vi "11_1.vi"() -> ()   [LabVIEW 2018]
uses:
  <userlib>/_OpenG.lib/array/array.llb/Search 1D Array (String)__ogtk.vi
panel:
  out "Occupied Seats":i32
  in  "Input":string="LLLLLLLLLLLLLLLLLLLLLLLLL.LLLLL..LLLLLLLLLLLL.LLL..LLLLLLLLLLLLLL.LL.LLLLL.LLLLLLLLL.LLLLLLLLLLLLL\nLLLLLLL.LLLLLLL.LLLLLLLLL.LLLLL.LLLL.LLLLLLLL.LLLLLLLLL.LLLL.LLLLLLLLLLLLLLLLLLLLLL..LLLLLLL..LLLL\nLLLLLL.LLLLLLLLLLLLLLLLLL.LLLLL.LLLLLLLLL.LLL.LLLLLLLLLLLLLL.LLLLLLL..LLLLLLLLLLLLLLLLLLLLLL.LLLLL\nLLLLLLL.LLLLLLLLLLLLLLLLLLLLLLL.LLLL.LLLLLLLLLLLLLLLLLLLL.LLLLLLLLLLLLLLL..LLLLLLLLL.LLLLLLL..LLLL\n.LLL.LL.LLLLLLL.LLLLLLLLL.LLLLLLLLLLLLLLLLLLLLLLLLLLLLLLLLLL.LLLLLLL.LLLLL.LLLLLLLLL.LLLLLLLLLLLLL\nLL.LLLL.LLLLLLLLLLLLLLLLL.LLLLL.LLLL.LLLLLLLLLLLLL.LLL.LLLLLLLLLLLLL.LLLLLLLLLLLLLLL.LLLLLLL.LLLLL\n......L........LLL....L.L......L.LL...L.....L.LL..L..L..L..LLL..LL......L...L.LL.L.L....L.........\nLLLLLLL.LLLLLLL.LLLLLLLLL.LLLLLLLLLL.LLLLLLLLL.LLL.LLLLLLLLL.L.LLLLL.LLLLL.LLLLLLLLL.LLLLLLL.LLLLL\nLLLLLLLLLLLLLLL.LLLLLLLLL.LLLLL.LLLL.LLLLLLLLLLLLLLLLLLLLLLL.LLLLLLL.LLLLL.LLLLLLLLLLLLLLLLL.LLLLL\nLLLLLLL.LLLLLLL.LLLLLLLLL.LLLLL.LLLL.LLLLLLLL.LLLL.LLLLLL.LL.LLLLLLL.LLLLLLLLLLLLLLL.LLLLLLL.LLLLL\nLLLLLLLLLLLLLLL.LLLLLLLLL.LLLLL.LLLL..LLLLLLL.LLLLLLLLLLLLLL.LLL.LLL..LLLL.LLLLLLLLL.LLLLLLL.LLLLL\nLLLLLLL.LLL.LLLLLLL.LLLLL.LLLLL.LLLL.LLLLLLLL.LLLL.LLLLLLLLLLLL.LLLL.L.LLL.LLLLLLLLLLLLLLLLL.LLLLL\nLLLLL.L.LLLLLLL.LLLLLL.LL.LLLLL.LLLL.LLLLLLLL.LLLL.LLLLLLLLL.L.L..LLLLLLL.LLLLLLLLLL.LLLLLLLLLLLLL\n.L....LLLL.LL.LL..L.L.L.L.LL..L..L.LLLLLL.L.LLLL.L.L..LL...L..L..LLL.....L........LL.L..L..L..L..L\nLLLLLLL.LLLLLLL.LLLLL.LLL.LLLLLLLLLL.LLLLL.LLLLLLL.LLLLLLLLLLLLLLLLLLLLLLL.LLLLLLLLL.LLLLLLLLLLLLL\nLLLLLLLLLLLLLLLLLL.LLLLLLLLLLLL..LLLLLLLLLLLL.LLLL.LLLLLLLLL.LLLLLLL.LLLLLLLLLLLLLLLLLLLLLLL.LLLLL\nLLLLLLL.LL.LLLL.LLLLLLLLLLLLLL.LLLLLLLL.LLLLLLLLLLLLLLLLLLLL.LLLLLLL.LLLLLLLLLLLLLLLLLLLLLLL.LLLLL\nLLLLLLL.LLLLLLL.LLLLLLLLL.LLLLL.LLLLLLLLLLLLL.LLLLLLLLLLLLLLLLLLLLLL.LLLLL.LLLLLLLLL.LLLLLLL.LLL.L\nLLLLLLLLLLLLLLL.LLLLLLLLL.LLLLLLLLLL.LLLLLLLLLLLLL.LLLLLLLLL.LLLLLLL.LLLLLLLL.LLLLLLLLLLL.LL.LLLLL\n.....L..L...L.L.L..........L..LLLL....L..L.L..LLLL...L..L....L.LL.L....L.L.L....LL.L..L......LLL.L\nLLLLLLL.LLLLLLL.LLLLLLLLLLLLLLLLLLLL.LLLLLLLLLLLLL.LLLLLLLLLLLLLLLLL.LLLLL.LL.LLLLLL.LL.LLLL.LLLLL\nLLLLLLL.L.LLLLLLLLLL.LLLL.L.LLLLLLLLLLLLLLLLLLLLLL.LLLLLLLLL.LLLLLLLLL.LLLLLLLLLLLLL.LLLLLLLLLLLLL\nLLLLLLL.LLLLLLL.LLLLLLLLL.LLLLL.LLLLLLLLLLLLL.LLLL.LLLLLLLLLLLLLLLLL.LLLLLLLLLLLL.LLLLLLLLLL.LLLLL\nLLLLLLL.LLLLLLLLLLLLLLLLL.LLLLL.L.LL.LLLLLLLLLLLLL.LLLLLLLLL.LLLL.LLLLLLLLLLLLLLL.L..LLLLLLLLLLL.L\nLLLLLLL.LLLLLLLLLLLLLLLLL.LLLLLLLLLL.LLLLLL.L.LLLL.L.LLLLLLLLLLLLLLL.LLLLLLLLLLLLL.L.LLLLLLLLLLLLL\nLLLLLLLLLLLLLLL.LLLLLL.LL.LLLLL.LLLLLLLLLLLLLLLLLLLLLLLLLLLL.LLLLLLL.LLLLL.LLLLLLLLL.LLLLLLL.LLLLL\nLLLLLLL.LL.LLLLLLLL.LLLLL.LLLLL.LLLL.LLLLLLLL.LLLLLLLLLLLLLL.LLLLLLL.LLLLL.LLLLLLL.L.LLLLLLL.LLLLL\nL.LLLLL.LLLLLLL.LLLLLLLLL.LLLLL.LLLLLLLLLLLLL.LLLLLLLLLLLLLL.LLLLLLL.LLLLLLLLLLLLLLL.LLLLLLLLLLLLL\nLLLLLLLLLLLLLLLLLLLLLLLLL.LLLLL.LLLLLLLLLLLLLLLLLL.LLLL.LLLL.LLLLLLL.LLLLLLLLLLLLLLLLLLLLLLLL.LLLL\n..L...L...L......L.LLLL.....LLL.L.LLLLLL.L.L.L..L.L.......L.L..L...L.L.L....LL...L.LL......LL.L.L.\nLLLLLLL.LLLLLLL.L.LLLLLLL.LLLLL.LLL.LLLLLLLLL.LLLLLLLLLLLLLL.LLLLLLL.LLLLL.LLLLLLLLL.LLLLLLL.LLLLL\nLLLLLLL.LLLLLLL.LLLLLLLLLLLLLLL.LLLLLLLLLLLLL..LLL.LLLLLLLLLLLLLLLLL.LLLLL.LLLLLLLLL.LLLLLLL.LLLLL\nLLLLLLL.LLLLLLLLLLLLLLLLL.LLLLL.LLLLLLLLLLLLLLLLLL.LLLLLLLLL.LLLLLLL.LLL.L.LLLLL.LLLLLLLLLLL.LLLLL\nLLLLLLL.LLLLLLL.LL.LLLLLL..LLLL.LLLLLLLLLLLLLLLLLLLLLLLLLLLLLLLLLLLL.LLLLL..LLLLLLLL.LLLL.LL.LLLLL\nLL.LLLL.LLLLLLLLL.LLLLLLL.LLLLLLLLLLLLLLLLLLLLLLLL.L.LLLLL.LLLLLLLLLLLLLLLLLLLLLLL.L.LLLLLLL.LLLLL\nLLLLLLL.LLLLLLL.LLLLLLLLL.LLLLL.LLLL.LLLLLLLL.LLLL.LLLLLL.LL.LLLLL.L.LLLLL.LLLLLLLLLLLLLLLLLLLLLLL\nLLLLLLL.LLL.LLL.LLLLLLLLLLLLLLL.LLLL.LLLLLLLL.LLLLLLLLLLLL.LLLLLLLLLLLLLLL.LLLLLLLLL.LLLLLLL.LLLLL\nL.L.......L.L....LL......LL.LL...LL..L...........L.....LLL....L..LL.LL.L.L.LL.......L.L...L....L..\nLLLLLLL.LLLLLLLLLLLLLLLLL.LLLLL.LLLL.LLLLLLLLLLLLL.LLLLLLLLL.LLLLLLL.LL.LL.LLLLLLLLLLLLLLLLL.LLL.L\nLLLLLLL.LLLLLLLLLLLLLLLLLLLLLLL.LLLL.LL.LLLLLLLLLL.LL.LLLLLL.LLLLLLLLLLLLL.LLLLLLLLLLLLLLLLLLLLLLL\nLLLLLLL.LLLLLLL.LLLLLLLLL.LLLLL.LLLL..LLLLLLLLLLLL.LLLLLLLLLLLLLLLLL.L..LL.LLL.LLLLLLLLLLLLLLLLLLL\nLLLLLLLLLL.LLLLLLLLLLLLLLLLLLLL.LLLL.LLLLLLLLLLLLL.LLLLLLLLLLLLLLLLLLLLLLL.LLLLLLLLL.LLLLLLL.LLLLL\nLLLLLLLLLL.LLLL.LLLLLLL.LLL.LLLLLLLL.LLLLLLLLLLLLL.LLLLLLLLL.LLLLLLLLLLLLLLLLLLLLLLLLLLLLLLL.LLLLL\nL.LLLLLLLLLLLLL.LL.LLLLLL.LLLLL.LLLL.LLLLLLLL.LLLLLLLLLLL.LL.LLLL.LLLLLLLLLL.LLLLLLL.LLLLLLL.LLLLL\n...LL.L..LL...L.......L.LL.......LL.LLL.L.LLL...L..LLL.L...L.......LL.LL.LL.L..LL........L.......L\nLLLLLLL.LLLLLLL.LLLLLLLLL.LLLLL.LLLL.LLLLLLLL.LLLLLLLLLLLLLL.LLLLLLL.LLLLL.LLLLLLLLLLLLLLLLL.LLLLL\nLLLLLLL.LLLLLLL.LLLLLLLLLLLLLLL.LLLL.LLLLLLLL.LLLLLLLLL.LLLL.LLLLLLL.LLLLL.LLLLLLLLLLLLLLLLLLLLLLL\nLLLLLLL.LLLLLLLLLLLLLLLLL.LLLLL.LLLLLLLLLLLLL.LLLL.LLLLLLLLL.LLLLL.L..LLLL.LLLLLLLLL.LLLL.LLLLLLLL\nLLLLLLLLLLLLLLL.LLLLLLLLLLLLLLL.LLLL.LLLLLLLL.LLLL..LLLLLLLLLLLLLLL..LL.LL.L.LLL.LLL.LLLLLLL.LLLLL\nLLLLL..LLLL.LLLLLLLLLLLLL.LLLLLLLL.L.LLLLLLLL.LLLL.LLLLLLLLL.L.LLL.LLLLLLL.LLLLLLLLL.LLLLLLLLLLLLL\nLLLLLLLLLLLLLLLLLLLLLLLLLLLLLLL.LLLL.LLLLLLLL.LLLL.LLLLLLLLLLLLLLLLLLLLL.L.LLLLLLLLL.LLLLL.L.LLLLL\n.LLLLLL.LLLLLLL..LLLLLLLL.LLLLLLLLLLLLLLLLLLL.LLLLLLLLLLLLLLLLLLLLLLLLLLLL.LLLLLLLLL.LLLLLLL.LLLLL\nLLLLLLL.LLLLLLLLLLL.LLLLLLLLLLLLLLL.LLLLLLLLLLLLLLLLLLLLLLLL.LLLLLLL.LLLLLLLLLLLLLLLLLLLLLLL.LLLLL\n..LL....L..........LL..L....L.LL...L.L...L.L...LLL..LL....LL.L.L.LLLL...L.L.......L.....LL........\nLLLLLLL.LLLLLLL.LLLLLLLLLLLLLLLLLLLL.LLLLLLLL.LLLLLLLLLLLLLL.LLLLLLLLLLLLLLLLLLLLLLL.LLLLLLL.LL.L.\nLLLLLLL.LLLL.LL.LLL.LLLLL.LLLLL.LLLL.LLLLLLL.LLLLL.LLLLLLLLLLLLLLLLL.LLLLLLLLLLLLLLL.LL.LLLLLLL.LL\nLL.LLLLLLLLLL.LLLLLLLLLLL.LLLLL.LLLL.LLLLLLLL.LLLL.LLLLLLLLL.LLL.LLL.LLLLL.LLLLLLLLL.LLLLLLL.LLLLL\nLLLLLLLLLLLLLLLL.LLLLLLLLLLLLLL.LLLL.LLLLLLLL.LLLLLLLLLLLLLL.LLLLLLL.LLLLL.LLLLLLLLL.LLLLLLL.LLLL.\nLLLLLLLLLLLLLLL.LLLLLLLL.LLLLLL.LLLL.LLLLLLLLLLLLL.LLLLLLLLL.LLL.LLL.L.LLLLLLLLLLLLLLLLLLLLL.LLLLL\nLLLLLLL.LLLLLLL.LLLLLLL.L.LLLLL.LLLL.LLLL.LLL.LLLLLLLLLL.LLLLLLLLLLL.LLLLL.LLLLLLLLL.LLLLLLL.LLL.L\nLLLLLLL.LLLLLLL.LLLLLLLLLLLLLLL.LLLL.L.LLLLLLLLLLL.LLLLLLLLL.LL.LLLL.LLLLLLLLLLLLLLL.LLLLLLLLLLLLL\nLLL.LLL.L.LLLLL.LLLLLLLLL.LLLLL.LLLL.LLLLLLLL.LLLL.LLLLLLL.L.LLLLLLLLL.LLL.LLLLLLLLLLLLLLLLLLLLLLL\n..LLL.LL.....LL...LL..L..LLL...........LL...........L.....L.......L..LLLLL......L......LL..L...L.L\nLLLLLLL.LLLLLLL.L.LLLLLLLLLL.LL.LLLL.LLLLLLLLLLLLL.LLLLLLL.L.LLLLLLLLLLLLLLLLLLLLLLLLLLLLLLL.LLLLL\nLLLLLLLLLLLLLLL.LL..LL.LLLLLLLL.LLLL.LLLLLLLLLLLLLLLLLLLLLLLLLLLLLLL.LLLLL.LLLLLLLLL.LLL.LLL.LLLLL\nLLLLLLL.LLLLLLL.LLLLLLLLL.LLLLL.LLLLLLLLLLLLL.LLLL.LLLLLLLLL.LLLLLLL..LLLL.LLLLLLLLLLLLLLLLLLLLLLL\nLLLLLLLLLLLL.LLLLLLLLLLLLLLLLLL.LLLLLLLLLLLLL.LLLL.LLLLLLLLL.LLLLLLLLL.LLLLLLLLLLLLLLLLLLLLL.LLLLL\nLLLLLLLLLLLLLLL.LLLLLLLLL.LLLLL.LLLLLLLLLLLLL.LLLLLLLLL.LLLL.LLLLLLL.LLLLLLLLLLLLLLL.LLLLLLLLLLLLL\nLLLLLLL.LLLLLLL.LLLLLLLLL.LLLLL.LLLL.LL.LLLLL.LLLL.LLLLLLLLL.LLLLLL.LLLLLL.LLLLLLLLL.LLLLLLL.L.LLL\nLLLLLLLLLLLLLLLLLLLLLLLLLLLLLLLLLLLL.LLLLLLLL.LLL..LLLLLLLLL.LLLLLLL.LLLLL.LLLLLLLLL.LLLLLLL..LLLL\nLLLLLLL.LLLLLLLLL.LLLLLLLLLLLLL.LLLL.LLLLLLLLLLLLL.LLLLLLLLL.LLLLLLLLLLLLL.LLLLLLL.LL.LLLLLLLLLLLL\nLLLLLLLLLLLLLLL.LLLLLLLLLLLLLLL.LLLL.LLLLLLLL.LLLL.LLLLLLLLL.LLLLLLL.LLLL..LLLLLLLLLLLLLLLLL.LLLLL\n.......L...LLL.L....L.LL......L.L...L...LL.LL...L...L..L.L.LL.........L.L..L.L.L.......L..L.....L.\nLLLLLLLLLLLLLLL.LLLLLLLLL.LLLLLLLLLL.LLLLLLL..LLLLLLLLLLLLL..LLLLL.LLLLLLL.LLLLLLLLL.LLLLLLLLLLLLL\nLLLLLLLLLLLLLLL.LLLLLLLLL.LLLLL.LLLL.LLLLLLLLLLLLL.LLLLLLLLL.LL.LLLLLLLLLL.LLLLLLLLLLLLLLLLL.LLLLL\nLLLLLLL.LLLLLLL.LLLLLLLLLLLLLLLLLLLLLLLLLLLLL.LL.LLLLLLLLLLLLLLLLL.L.LLLLL.LLLLLLLLL.LLLLLLL.LLLLL\nLLLLLLL.LLLLLLL.LLLLLLLLL.LLLLL.LLLLLLLLLLLLLLLLLL.LLLLL.LLL.LLLLLLLLLLLLL.L.LLLLLLL.LLLLLLLLLLLLL\nLLLLLLL.LLL.LLL.LLLLLLLLL.LLLLL.LLLLLLLLLLLLL.LLLL.LLLLLLLLL.LLLLLLL.LLLLL.LLLLLLLLLLLLLLLLL.LLLLL\nLLLLLL..LL.LLLLL.LLLLLLLL.L.LLL.LLLL.LLLLLLLLLLLLLLLL..LLLLL.LLLLLLLLLLLLLLLLLLLLLLLLLLLLLLLLLLLLL\n.LLLL.L.LLLLLLL.LLLLLLLLL.LLLLLLLLLL..LLL.LLL.LLLL.LLLLLLLLL.LLLL.LL.LLLLL.LLLLLLLLL.LLLLLLL..L.LL\nLLLLLLL.LLLLLLLLLLLLLLLLLLLLLLLLLLL..LL.LLLLLLLLLL.LL.LLLLLL.LLLLL.L.LLLLL.LLLLLL..LLLLLLLLL.LLLLL\n..L...L..L..L.L..LL.L.LLL.LLL.L....L..LL.....L....LL...L.L.L.L...L.L.....LLL......L...LL.L.......L\nLLLLLLLLLLLLLLL.LLLLLLLLL.LLLL.LLLLL.LLLLLLL.LLLLL..LLLLLLLLLLL.L.LL.LLLLLLLLLLLL.LL.LLL.LLL.LLLLL\nLLLLLLL.LLLLLL..LLLLLLLLL.LLLLLLLLLL.LLLLLLLL.LLLL.LLLLLLLLL.LLLLLLL.LLLLLLLLLLLLLLL.LLLLLLL.LLLLL\nLLLLLLL..LLLLLL.LLLLLLLLLLLLLLL.LLLL.LLLLLLLL.LLLL.LLLLLLLLL.LLLLLLL.LLLLL.LLLLLLLLLLLLLLLLLLLLLLL\nLLLLLLLLLLLLLLLLLLLLLLLLLLLLLLL.LLLL.LLLLLLLL.LLLL.LLLLLLLLLL.LLLLLL.LLLLLLLLLLLLLLL.LLLLLLL.L.LLL\nLLLLLLL.LLLLLLLLLLLLLLLLL.LLLLL.LLLL.LLLLLLLL.LLLL.LLLLLLLLLLLLLLLLL.LLLLLLLLLLLLLLL.LLLL.LL.LLLLL\n..L..LL.L.L...LL...L.LL.LL....L.L.L.LLL...LL.LL...L...L...LLLLLL.LLL...L.L.LL................LL.L.\nLLLLLLLLLLL.LLL.LLLLLLLLL.LLLLL.LLLLLLLLLLLLL.LLL.LLLLLLLLLL.LLLLLLL.LLLLLLLLLL.LLLL.LLLLLLLLLLLLL\nLLLLLLL.LLLLLLLLLLLLLLLLL.LLLLLLLLLL.LLLLLLLLLLLLL.LLLLLLLLL.LLLLLLL.LLLLL.LLLLLLLLL.LLLLLLLLLLLLL\nLLLLLLL.LLLLL.L.LLL.LLLLLLLLLLLLLLLLLLLL.LLLLLLLLL.LLLLLLLLL.LLL.LLL.LLLLL.LLLLLLLLLLLLLLLLLLLLLLL\nLLLLLLL.LLLLLLL.LLLLLLLLL.L.LLL.LL.LLLLLLLL.L.LLLL.LLLLLLLLL.LLLLLLLLLLLLLLLLLLLLLLL.LLLLLLLLLLLLL\n.LL.LLL.LLLLLLL.LLLLLLLLL.LLLLL.LLLLLLLLLLLLL.LLLL.LLLLLLLLL.LLLLLLLLLLL.L.LLLLLLLLLLLLLLLLL.LLLLL\nLLLLLLL.LLLLLLLLLLLLLLLLL.LLLLLLLLLL.LLLLLLLL.LL.LLLL.LLLLLL.LLLLLLLLLLLLLLLLLLLLLLL.LLLLLLLLLLLLL\nLLLL.LL.LLLLLLL.LLLLLLLLL.LLLLL.LLLLLLLLLLLLLLLLLL.LLLLLLLLLLLLLLLLL.LLLLLLLLLLLLLLL.LLLLLLL.LLLLL\nLLLLLLLLLLLLLLLLLLLLLLLLL.LLLLL.LL.LLLLLLLLLL.LLLL.LLLLLLLLL.LLLLLLL.LLLLL.LLLLLLL.LLLLLLLLL.LLLLL\nLLLLLLL.LLLLLLL..LLLLLLLLLLLLLLLLLLL.LLLLLLLLLLLLL.LLLLLLLLL.LL.LLLL.LLLLL.LLLLLLLLL.LLLLLLL.LLLLL\n"
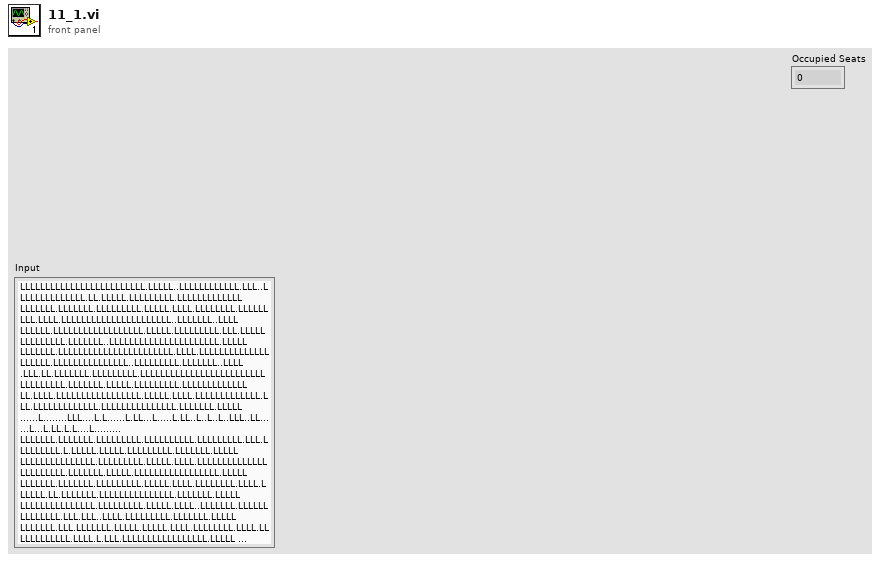
[diagram p1: front panel]
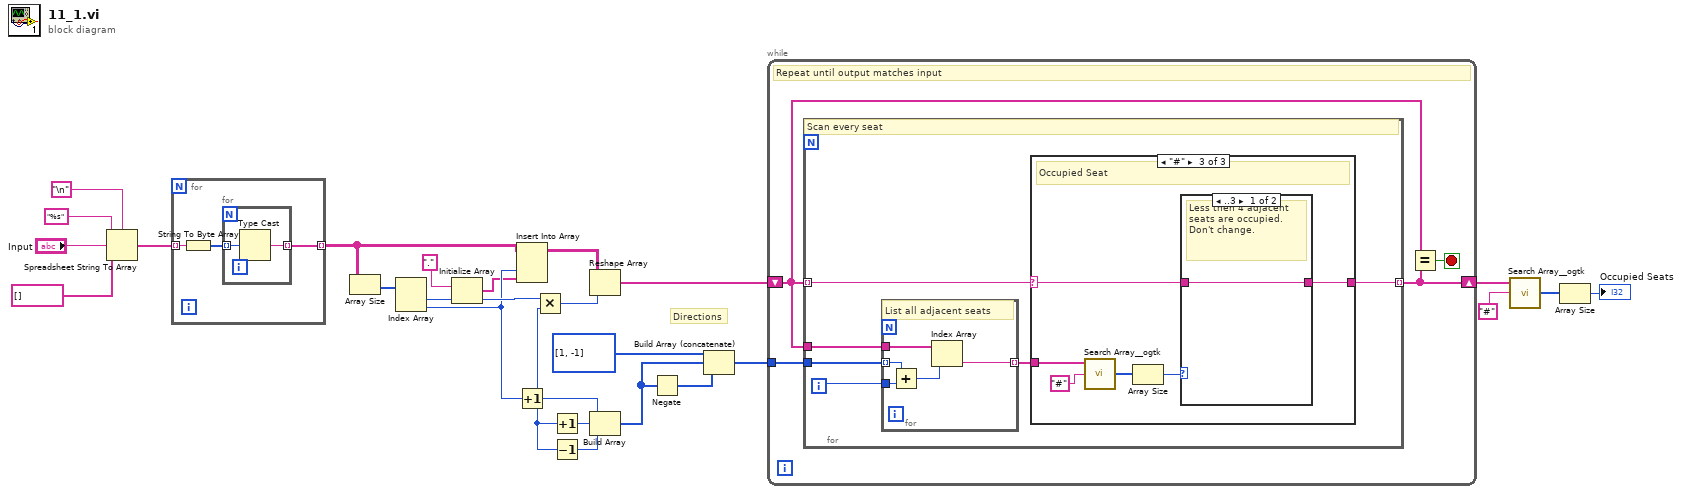
[diagram p0: block diagram]
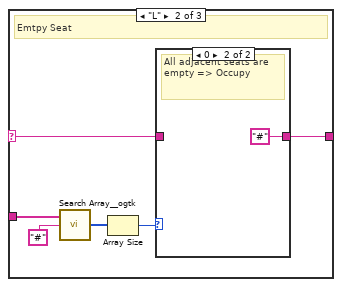
[diagram p3: hidden frame]
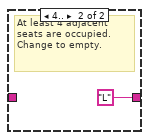
[diagram p5: hidden frame]
diagram:
  # "Directions"
  n1 = Spreadsheet String To Array(delimiter (Tab)="\n", format string="%s", spreadsheet string="Input", array type (2D Dbl)=string[] []) -> (array=w22:string[])
  n2 = for {
    tunnel: w22 -> [w28] mode=indexing
    tunnel: [w26] -> w18 mode=indexing
    n3 = String To Byte Array(string=w28) -> (unsigned byte array=w27:u8[])
    n4 = for {
      tunnel: w27 -> [w30] mode=indexing
      tunnel: [w29] -> w26 mode=indexing
      n5 = Type Cast(x=w30) -> (*(type *) &x=w29:string)  [unwired: 1 in]
    }
  }
  n6 = Array Size(array=w18) -> (size(s)=w20:i32[])
  n7 = Index Array(array=w20) -> (element #1=w17:i32, element #2=w14:i32)  [unwired: 2 in]
  n8 = Initialize Array(".", w17) -> (w2:string[])
  n9 = Insert Into Array(array=w18, index (col)=w14, new element=w2) -> (w15:string[][])  [unwired: 1 in]
  n10 = Increment(x=w14) -> (x+1=w1:i32)
  n11 = Multiply(x=w17, y=w1) -> (x*y=w16:i32)
  n12 = Increment(x=w1) -> (x+1=w12:i32)
  n13 = Decrement(x=w1) -> (x-1=w11:i32)
  n14 = Reshape Array(w15, w16) -> (w7:string[])
  n15 = Build Array(w1, w12, w11) -> (w10:i32[])
  n16 = Negate(x=w10) -> (-x=w9:i32[])
  n17 = Build Array (concatenate)(i32[] [1, -1], w10, w9) -> (w8:i32[])
  n18 = while {
    shift-right: [w33] -> w6
    shift-left: w7 -> [w32]
    tunnel: w8 -> [w34]
    stop <- w31 stop-if-true
    # "Repeat until output matches input"
    n19 = for {
      tunnel: w32 -> [w38]
      tunnel: w34 -> [w36]
      tunnel: w32 -> [w40] mode=indexing
      tunnel: [w39] -> w33 mode=indexing
      i -> [w35]
      # "Scan every seat"
      n20 = for {
        tunnel: w38 -> [w45]
        tunnel: [w44] -> w37 mode=indexing
        tunnel: w36 -> [w43] mode=indexing
        tunnel: w35 -> [w42]
        # "List all adjacent seats"
        n21 = Add(x=w43, y=w42) -> (x+y=w41:i32)
        n22 = Index Array(array=w45, index=w41) -> (element=w44:string)
      }
      n23 = case shown="\"#\"" w40 {
        selector: w40 -> [w46 w51 w59]
        tunnel: [w46 w52 w60] -> w39
        tunnel: w37 -> [_ w49 w55]
        frame ".", Default {
          # "Floor doesn't change"
        }
        frame "L" {
          # "Emtpy Seat"
          n24 = call-poly <userlib>:"Search Array__ogtk.vi"("Array"=w49, "Element Data"="#") -> ("Indices of Elements"=w50:i32[])  [unwired: 7 in]
          n25 = Array Size(array=w50) -> (size(s)=w47:i32)
          n26 = case shown="0" w47 {
            tunnel: [w53 "#"] -> w52
            tunnel: w51 -> [w53 _]
            frame Default {
              # "At least 1 adjacent seat is occupied.\nDon't change"
            }
            frame 0 {
              # "All adjacent seats are empty => Occupy"
            }
          }
        }
        frame "#" {
          # "Occupied Seat"
          n27 = call-poly <userlib>:"Search Array__ogtk.vi"("Array"=w55, "Element Data"="#") -> ("Indices of Elements"=w57:i32[])  [unwired: 7 in]
          n28 = Array Size(array=w57) -> (size(s)=w56:i32)
          n29 = case shown="..3" w56 {
            tunnel: [w61 "L"] -> w60
            tunnel: w59 -> [w61 _]
            frame ..3 {
              # "Less then 4 adjacent seats are occupied.\nDon't change."
            }
            frame 4.. {
              # "At least 4 adjacent seats are occupied.\nChange to empty."
            }
          }
        }
      }
    }
    n30 = Equal?(x=w32, y=w33) -> (x = y?=w31:bool)
  }
  n31 = call-poly <userlib>:"Search Array__ogtk.vi"("Array"=w6, "Element Data"="#") -> ("Indices of Elements"=w4:i32[])  [unwired: 7 in]
  n32 = Array Size(array=w4) -> (size(s)=→"Occupied Seats":i32)
